vi "testMessage.vi"() -> (0 "error out":errorcluster)   [LabVIEW 2019, in "AssertionTest.lvlib" / "AssertCount.lvlib"]
uses:
  AssertCount.lvlib
  AssertionTest.lvlib
  Assertion/Assertion.lvlib
  Error/Error.lvlib
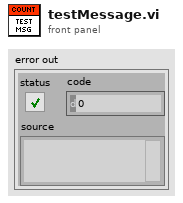
[diagram p1: front panel]
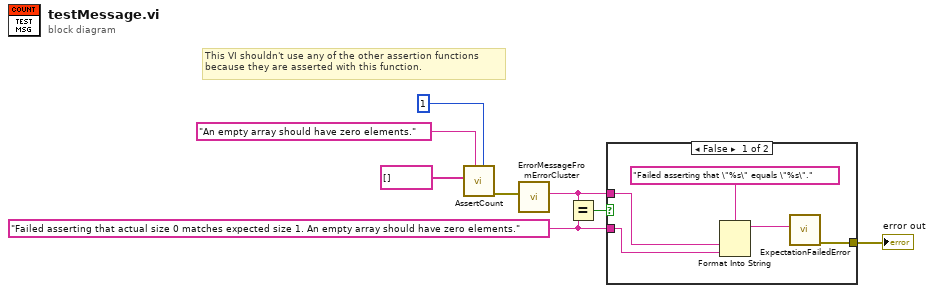
[diagram p0: block diagram]
diagram:
  w7 = "Failed asserting that actual size 0 matches expected size 1. An empty array should have zero elements." ("y")
  # "This VI shouldn't use any of the other assertion functions\nbecause they are asserted with this function."
  n1 = call "AssertCount.vi"("Expected"=1, "Message (\"\")"="An empty array should have zero elements." ("Message (\"\")"), "Haystack"=string[] []) -> ("error out"=w6:errorcluster)  [unwired: 8 in]
  n2 = call "ErrorMessageFromErrorCluster.vi"("Error"=w6) -> ("Error Message"=w5:string)  [unwired: 10 in]
  n3 = Equal?(x=w5, y=w7) -> (x = y?=w8:bool)
  n4 = case shown="False" w8 {
    tunnel: w5 -> [w12 _]
    tunnel: w7 -> [w11 _]
    tunnel: [w9 _] -> w1
    frame False {
      n5 = Format Into String(format string="Failed asserting that \"%s\" equals \"%s\".", w12, w11) -> (resulting string=w10:string)  [unwired: 2 in, 1 out]
      n6 = call "ExpectationFailedError.vi"("Message"=w10) -> ("error out"=w9:errorcluster)  [unwired: 10 in]
    }
    frame True {
    }
  }
  "error out" <- w1
